vi "Wait for Result.vi"(6 "Last request":bool, 8 "error in (no error)":errorcluster, 11 "Instrument Recorder in":refnum<class "Instrument Actor.lvclass">) -> (0 "error out":errorcluster, 3 "Instrument Recorder out":refnum<class "Instrument Actor.lvclass">)   [LabVIEW 2016, in "Instrument Actor.lvclass"]
uses:
  Instrument Actor.lvclass
  C:/github/LabActor/Worker/Worker.lvclass
  C:/github/LabActor/Template Module/Template Module.lvclass
  C:/Program Files/National Instruments/LabVIEW 2016/vi.lib/ActorFramework/Actor/Actor.lvclass
  Worker/Worker.lvclass/Worker.ctl
  Template Module/Template Module.lvclass/Template Module.ctl
  NHMFL_Core/Libraries/Instruments/Results/Acquired Result/Acquired Result.lvclass/Acquired Result.ctl
  <vilib>/ActorFramework/Actor/Actor.lvclass/Actor.ctl
  <vilib>/ActorFramework/Message Enqueuer/Message Enqueuer.lvclass/Message Enqueuer.ctl
  Instrument Actor.lvclass/Instrument Actor.ctl
  Pulse Recorders/Pulse Recorder Messages/Wait for Data Msg/Wait for Result Msg.lvclass/Wait for Result Msg.ctl
  Template Module/Read Reply to.vi
  Template Module/Read Name.vi
  NHMFL_Core/Libraries/Instruments/Results/Acquired Result/Write Sender.vi
  NHMFL_Core/Libraries/Instruments/Results/Acquired Result/Read Final.vi
  NHMFL_Core/Libraries/Instruments/Results/Acquired Result/Write Cycle count.vi
  Template Module/Read State.vi
  <vilib>/ActorFramework/Message Enqueuer/Init from Existing Queue.vi
  Pulse Recorders/Pulse Recorder Messages/Wait for Data Msg/Wait for Result Msg.lvclass
  C:/Program Files/National Instruments/LabVIEW 2016/vi.lib/ActorFramework/Message/Message.lvclass
  <vilib>/ActorFramework/Time-Delayed Send Message/Time-Delayed Send Message.vi
  Template Module Messages/Result Reply Msg/Result Reply Msg.lvclass
  <vilib>/ActorFramework/Message Enqueuer/Message Enqueuer.lvclass
  <vilib>/ActorFramework/Actor/Actor.lvclass
  NHMFL_Core/Libraries/Instruments/Results/Acquired Result/Acquired Result.lvclass
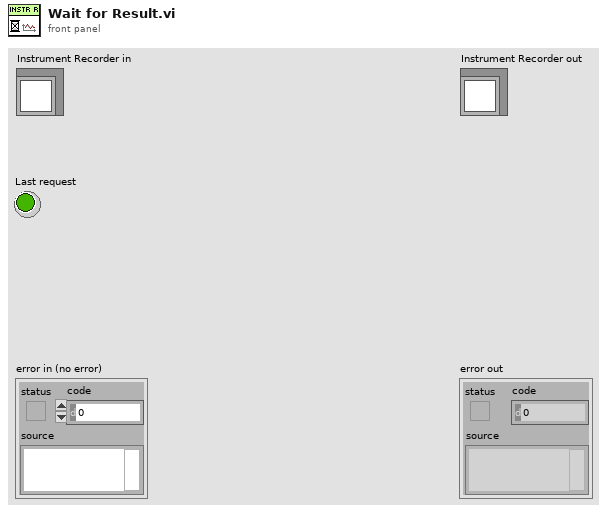
[diagram p1: front panel]
types:
  T1 = typedef "Worker State.ctl" = enum16{"Idle", "Starting", "Working", "Stopping"}
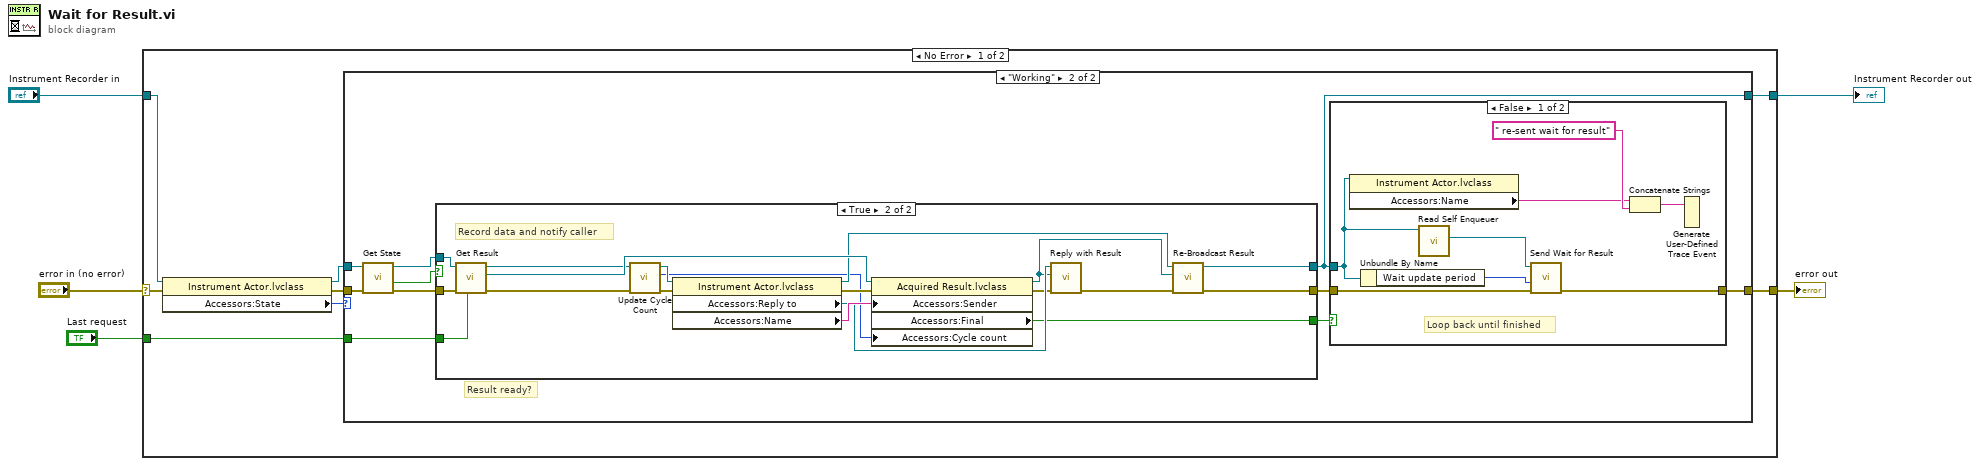
[diagram p0: block diagram]
diagram:
  n1 = case shown="No Error" "error in (no error)" {
    selector: "error in (no error)" -> [w13 w58]
    tunnel: [w11 w58] -> w4
    tunnel: [w12 w57] -> w2
    tunnel: "Instrument Recorder in" -> [w8 w57]
    tunnel: "Last request" -> [w10 _]
    frame No Error {
      n2 = property class="Instrument Actor.lvclass"(reference=w8, error in=w13) -> (reference out=w7:refnum<class "Instrument Actor.lvclass">, error out=w9:errorcluster, "Accessors:State"=w6:T1)
      n3 = case shown="\"Working\"" w6 {
        tunnel: w9 -> [w15 w25]
        tunnel: w7 -> [w14 w23]
        tunnel: [w14 w19] -> w12
        tunnel: [w15 w17] -> w11
        tunnel: w10 -> [_ w16]
        frame "Idle", Default {
        }
        frame "Working" {
          # "Result ready?"
          n4 = call-dynamic "Get State.vi"("error in (no error)"=w25, "Instrument Actor in"=w23) -> ("error out"=w24:errorcluster, "Result ready"=w21:bool, "Instrument Actor out"=w22:refnum<class "Instrument Actor.lvclass">)  [unwired: 5 in, 2 out]
          n5 = case shown="True" w21 {
            selector: w21 -> [w35 _]
            tunnel: w22 -> [w37 w56]
            tunnel: w24 -> [w36 w55]
            tunnel: [w36 w44] -> w18
            tunnel: [w37 w43] -> w19
            tunnel: [w35 w49] -> w20
            tunnel: w16 -> [_ w42]
            frame False {
            }
            frame True {
              # "Record data and notify caller"
              n6 = call-dynamic "Get Result.vi"("Last request"=w42, "error in (no error)"=w55, "Instrument Recorder in"=w56) -> ("error out"=w48:errorcluster, "Result"=w50:refnum<class "Acquired Result.lvclass">, "Instrument Recorder out"=w40:refnum<class "Instrument Actor.lvclass">)  [unwired: 6 in]
              n7 = call-dynamic "Update Cycle Count.vi"("error in (no error)"=w48, "Worker in"=w40) -> ("error out"=w41:errorcluster, "Cycle count out"=w38:i32, "Worker out"=w39:refnum<class "Instrument Actor.lvclass">)  [unwired: 7 in]
              n8 = property class="Instrument Actor.lvclass"(reference=w39, error in=w41) -> (reference out=w47:refnum<class "Instrument Actor.lvclass">, error out=w54:errorcluster, "Accessors:Reply to"=w52:refnum<class "Result Reply Msg.lvclass">, "Accessors:Name"=w53:string)
              n9 = property class="Acquired Result.lvclass"(reference=w50, error in=w54, "Accessors:Sender"=w53, "Accessors:Cycle count"=w38) -> (reference out=w46:refnum<class "Acquired Result.lvclass">, error out=w51:errorcluster, "Accessors:Final"=w49:bool)
              n10 = call-dynamic "Reply with Result.vi"("error in (no error)"=w51, "Result"=w46, "Result Reply Msg in"=w52) -> ("error out"=w45:errorcluster)  [unwired: 7 in, 1 out]
              n11 = call-dynamic "Re-Broadcast Result.vi"("error in (no error)"=w45, "Acquired Result.lvclass"=w46, "Measure Object in"=w47) -> ("error out"=w44:errorcluster, "Measure Object out"=w43:refnum<class "Instrument Actor.lvclass">)  [unwired: 7 in]
            }
          }
          n12 = case shown="False" w20 {
            tunnel: w19 -> [w29 _]
            tunnel: w18 -> [w31 w34]
            tunnel: [w30 w34] -> w17
            frame False {
              # "Loop back until finished"
              n13 = property class="Instrument Actor.lvclass"(reference=w29) -> ("Accessors:Name"=w27:string)  [unwired: 1 in, 2 out]
              n14 = Unbundle By Name(w29) -> ("Wait update period"=w32:i32)
              n15 = call <vilib>:"Read Self Enqueuer.vi"("Actor"=w29) -> ("Self Enqueuer"=w33:refnum<class "Message Enqueuer.lvclass">)  [unwired: 10 in]
              n16 = call "Send Wait for Result.vi"("error in (no error)"=w31, "Milliseconds To Wait"=w32, "Message Enqueuer"=w33) -> ("error out"=w30:errorcluster)  [unwired: 6 in, 2 out]
              n17 = Concatenate Strings(w27, " re-sent wait for result" ("string")) -> (w26:string)
              n18 = Generate User-Defined Trace Event(2:w26) -> ()  [unwired: 1 in]
            }
            frame True {
            }
          }
        }
      }
    }
    frame Error {
    }
  }
  "error out" <- w4
  "Instrument Recorder out" <- w2
